vi "write chassis object.vi"(8 "error in":errorcluster, 10 "chassis information":T1 {"product ID" format="%.0x"}, 11 "Chassis in":refnum<class "Chassis.lvclass">) -> (0 "error out":errorcluster, 3 "Chassis out":refnum<class "Chassis.lvclass">)   [LabVIEW 2014, in "SMI.lvlib" / "Chassis.lvclass"]
uses:
  Chassis.lvclass
  chassis information.ctl
  Chassis.lvclass/Chassis.ctl
  Device/write device class.vi
  Device/write serial number.vi
  Device/write product ID.vi
  Device/write product name.vi
  Device/write vendor name.vi
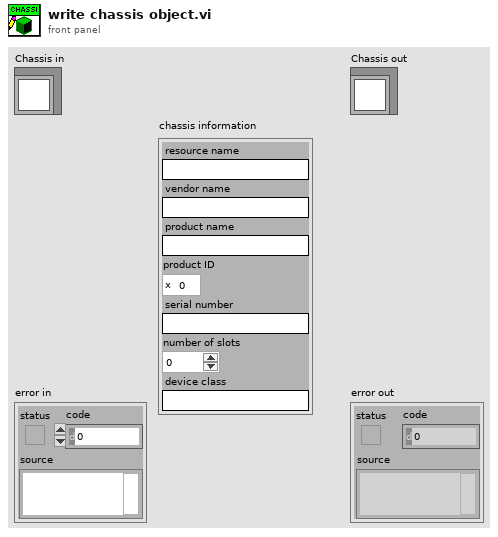
[diagram p1: front panel]
types:
  T1 = typedef "SMI.lvlib/Chassis.lvclass/chassis information.ctl" = cluster{"resource name":string, "vendor name":string, "product name":string, "product ID":u16, "serial number":string, "number of slots":i32, "device class":string}
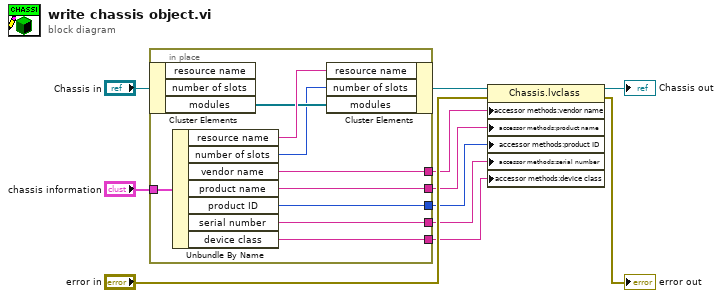
[diagram p0: block diagram]
diagram:
  n1 = in-place {
    in-place-border: "chassis information" -> [w20]
    in-place-border: [w16] -> w7
    in-place-border: [w15] -> w6
    in-place-border: [w14] -> w5
    in-place-border: [w13] -> w4
    in-place-border: [w12] -> w1
    n2 = in-place-cluster #1("Chassis in") -> ("modules"=w18:refnum<class "Module.lvclass">[])  [unwired: 2 out]
    n3 = Unbundle By Name(w20) -> ("resource name"=w19:string, "number of slots"=w17:i32, "vendor name"=w16:string, "product name"=w15:string, "product ID"=w14:u16, "serial number"=w13:string, "device class"=w12:string)
    n4 = in-place-cluster #1("resource name"=w19, "number of slots"=w17, "modules"=w18) -> (w10:refnum<class "Chassis.lvclass">)
  }
  n5 = property class="Chassis.lvclass"(reference=w10, error in="error in", "accessor methods:vendor name"=w7, "accessor methods:product name"=w6, "accessor methods:product ID"=w5, "accessor methods:serial number"=w4, "accessor methods:device class"=w1) -> (reference out=→"Chassis out":refnum<class "Chassis.lvclass">, error out=→"error out":errorcluster)
